vi "Initialize camera.vi"(8 "error in (no error)":errorcluster, 11 "Channel in":refnum<class "SPARC4_Channel.lvclass">) -> (0 "error out":errorcluster, 3 "Channel out":refnum<class "SPARC4_Channel.lvclass">)   [LabVIEW 2018, in "SPARC4_Channel.lvclass"]
doc: "Initialize the camera"
uses:
  SPARC4_Channel.lvclass
  Sim_CCD/Sim_CCD.lvclass
  Sim_Ixon_Ultra/Sim_Ixon_Ultra.lvclass
  C:/Users/Denis/Desktop/S4ACS/S4ACS/Sim_CCD/Sim_CCD.lvclass
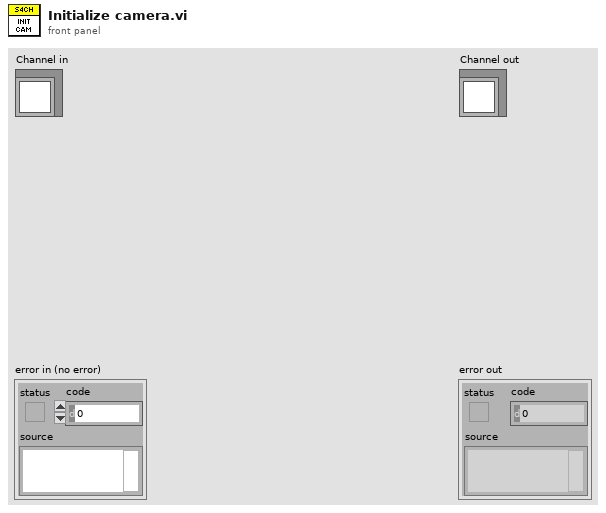
[diagram p1: front panel]
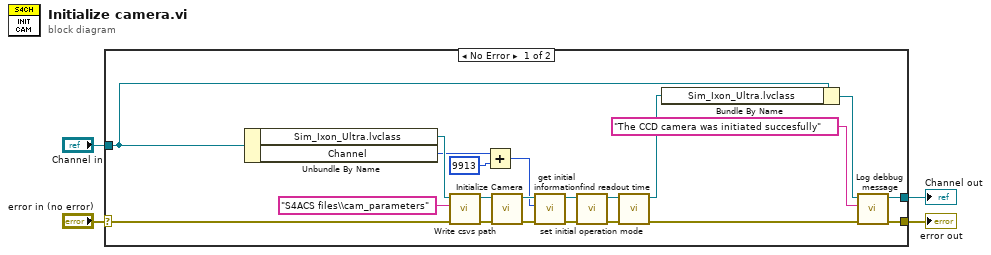
[diagram p0: block diagram]
diagram:
  n1 = case shown="No Error" "error in (no error)" {
    selector: "error in (no error)" -> [w12 w27]
    tunnel: [w19 w27] -> w3
    tunnel: [w20 w26] -> w1
    tunnel: "Channel in" -> [w25 w26]
    frame No Error {
      n2 = Unbundle By Name(w25) -> ("Sim_Ixon_Ultra.lvclass"=w9:refnum<class "Sim_Ixon_Ultra.lvclass">, "Channel"=w7:u8)
      n3 = call "Write csvs path.vi"("error in (no error)"=w12, "csvs path"="S4ACS files\\cam_parameters", "Simulated Camera in"=w9) -> ("error out"=w11:errorcluster, "Simulated Camera out"=w10:refnum<class "Sim_Ixon_Ultra.lvclass">)  [unwired: 7 in]
      n4 = Add(x=w7, y=u16 9913) -> (x+y=w5:u16)
      n5 = call-dynamic "Initialize Camera.vi"("error in (no error)"=w11, "CCDCamera in"=w10) -> ("error out"=w23:errorcluster, "CCDCamera out"=w24:refnum<class "Sim_Ixon_Ultra.lvclass">)  [unwired: 8 in]
      n6 = call-dynamic "get initial information.vi"("error in (no error)"=w23, "SERN"=w5, "Simulated_CCD_Camera in"=w24) -> ("error out"=w16:errorcluster, "Simulated_CCD_Camera out"=w13:refnum<class "Sim_Ixon_Ultra.lvclass">)  [unwired: 7 in]
      n7 = call-dynamic "set initial operation mode.vi"("error in (no error)"=w16, "Simulated_CCD_Camera in"=w13) -> ("error out"=w15:errorcluster, "Simulated_CCD_Camera out"=w14:refnum<class "Sim_Ixon_Ultra.lvclass">)  [unwired: 8 in]
      n8 = call-dynamic "find readout time.vi"("error in (no error)"=w15, "Simulated_CCD_Camera in"=w14) -> ("error out"=w18:errorcluster, "Simulated_CCD_Camera out"=w22:refnum<class "Sim_Ixon_Ultra.lvclass">)  [unwired: 8 in]
      n9 = Bundle By Name(cluster=w25, "Sim_Ixon_Ultra.lvclass"=w22) -> (w21:refnum<class "SPARC4_Channel.lvclass">)
      n10 = call "Log debbug message.vi"("error in (no error)"=w18, "String"="The CCD camera was initiated succesfully", "Channel in"=w21) -> ("error out"=w19:errorcluster, "Channel out"=w20:refnum<class "SPARC4_Channel.lvclass">)  [unwired: 7 in]
    }
    frame Error {
    }
  }
  "error out" <- w3
  "Channel out" <- w1
